vi "Update Btifle Path.vi"(7 "Bitfile Path Ref":refnum<vi>, 8 "error in (no error)":errorcluster, 11 "Bitfile Path":path) -> (0 "error out":errorcluster)   [LabVIEW 2025, in "I2C Bus Monitor UI.lvlib"]
uses:
  I2C Bus Monitor UI.lvlib
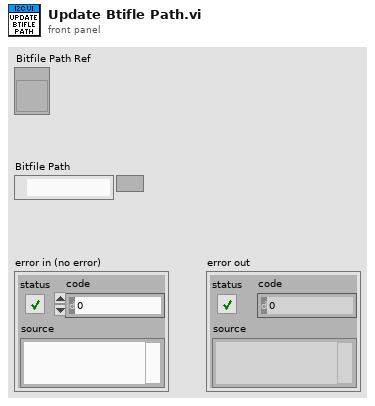
[diagram p1: front panel]
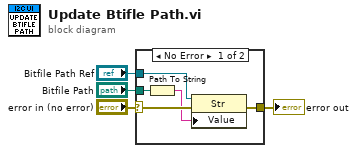
[diagram p0: block diagram]
diagram:
  n1 = case shown="No Error" "error in (no error)" {
    selector: "error in (no error)" -> [w8 w10]
    tunnel: [w9 w10] -> w4
    tunnel: "Bitfile Path" -> [w6 _]
    tunnel: "Bitfile Path Ref" -> [w5 _]
    frame No Error {
      n2 = Path To String(path=w6) -> (string=w7:string)
      n3 = property class="Str"(reference=w5, error in=w8, "Value"=w7) -> (error out=w9:errorcluster)  [unwired: 1 out]
    }
    frame Error {
    }
  }
  "error out" <- w4
